vi "Ext.vi"(8 "error in (no error)":errorcluster, 9 "Val":variant, 10 "Tag":u16, 11 "Square in":refnum<class "Rigol DG822 Square.lvclass">) -> (0 "error out":errorcluster, 1 "Parsed":variant, 3 "Square out":refnum<class "Rigol DG822 Square.lvclass">)   [LabVIEW 2021, in "Rigol DG822 UI.lvlib" / "Rigol DG822 Square.lvlib" / "Rigol DG822 Square.lvclass"]
uses:
  Rigol DG822 Square.lvclass
  Rigol DG822 UI/lib/controls.llb/WaveformExtCall.ctl
  Rigol DG822 UI/lib/controls.llb/WaveformParamTags.ctl
  Rigol DG822 Square.lvclass/Rigol DG822 Square.ctl
  Rigol DG822 UI/lib/controls.llb/AllWaveformDataCluster.ctl
  Rigol DG822 UI/lib/controls.llb/DataCluster.ctl
  Rigol DG822 UI/lib/controls.llb/FT Controls Cluster.ctl
  Rigol DG822 UI/lib/controls.llb/String Indicators Cluster.ctl
  General/Files/lvlibp/Actors.lvlibp/Actors/Actors/Actors.lvclass
  D:/LabVIEW/General/Files/lvlibp/Actors.lvlibp/Actors/Actors/Actors.lvclass
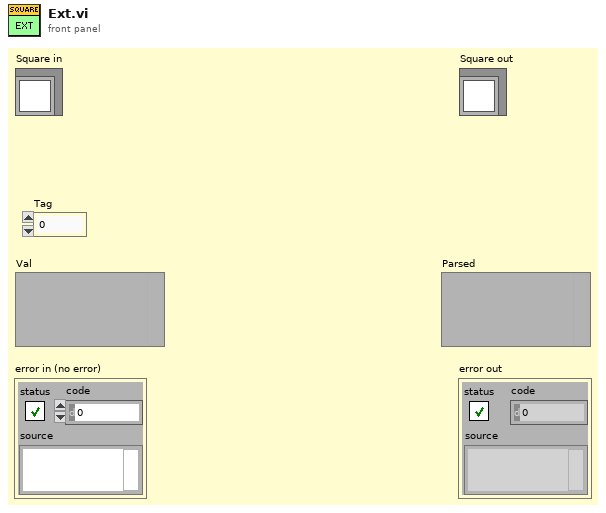
[diagram p1: front panel]
types:
  T1 = typedef "WaveformExtCall.ctl" = enum16{"Freq", "Period", "Ampl", "HighL", "Offset", "LowL", "Phase", "Duty", "Width", "RisEdge", "FallEdge", "Home", "InitData"}
  T2 = typedef "AllWaveformDataCluster.ctl" = cluster{"Data":T3, "F/T Ctrls":T4, "String Indcs":T5}
  T3 = typedef "DataCluster.ctl" = cluster{"Freq":cluster{"Freq":dbl, "FreqUnit":enum32{"No Selection", "MHz", "kHz", "Hz", "mHz", "uHz"}, "FreqUnitPrcs":dbl}, "Period":cluster{"Period":dbl, "PeriodUnit":enum32{"No Selection", "s", "ms", "us", "ns"}, "PeriodUnitPrcs":dbl}, "Ampl":cluster{"Ampl":dbl, "AmplUnit":enum32{"No Selection", "Vpp", "mVpp"}, "AmplUnitPrcs":dbl}, "HighL":cluster{"HighL":dbl, "HighLUnit":enum32{"No Selection", "V", "mV"}, "HighLUnitPrcs":dbl}, "Offset":cluster{"Offset":dbl, "OffsetUnit":enum32{"No Selection", "Vdc", "mVdc"}, "OffsetUnitPrcs":dbl}, "LowL":cluster{"LowL":dbl, "LowLUnit":enum32{"No Selection", "V", "mV"}, "LowLUnitPrcs":dbl}, "Phase":cluster{"Phase":dbl, "PhaseUnit":enum32{"°"}, "PhaseUnitPrcs":dbl}, "Duty":cluster{"Duty":dbl, "DutyUnit":enum32{"%"}, "DutyUnitPrcs":dbl}, "Width":cluster{"Width":dbl, "WidthUnit":enum32{"No Selection", "s", "ms", "us", "ns"}, "WidthUnitPrcs":dbl}, "RisEdge":cluster{"RisEdge":dbl, "RisEdgeUnit":enum32{"No Selection", "s", "ms", "us", "ns"}, "RisEdgeUnitPrcs":dbl}, "FallEdge":cluster{"FallEdge":dbl, "FallEdgeUnit":enum32{"No Selection", "s", "ms", "us", "ns"}, "FallEdgeUnitPrcs":dbl}}
  T4 = typedef "FT Controls Cluster.ctl" = cluster{"Freq/Period":bool, "Ampl/HighL":bool, "Offset/LowL":bool, "Duty/Width":bool}
  T5 = typedef "String Indicators Cluster.ctl" = cluster{"Freq-Period":string, "Ampl-HighL":string, "Offset-LowL":string, "Phase":string, "Duty-Width":string, "RisEdge":string, "FallEdge":string}
  T6 = typedef "WaveformParamTags.ctl" = enum16{"Freq", "Period", "Ampl", "HighL", "Offset", "LowL", "Phase", "Duty", "Width", "RisEdge", "FallEdge"}
  T7 = cluster{"Duty":dbl, "DutyUnit":enum32{"%"}, "DutyUnitPrcs":dbl}
  T8 = cluster{"Freq":dbl, "FreqUnit":enum32{"No Selection", "MHz", "kHz", "Hz", "mHz", "uHz"}, "FreqUnitPrcs":dbl}
  T9 = cluster{"Period":dbl, "PeriodUnit":enum32{"No Selection", "s", "ms", "us", "ns"}, "PeriodUnitPrcs":dbl}
  T10 = cluster{"Freq":cluster{"Freq":dbl, "FreqUnit":enum32{"No Selection", "MHz", "kHz", "Hz", "mHz", "uHz"}, "FreqUnitPrcs":dbl}, "Period":cluster{"Period":dbl, "PeriodUnit":enum32{"No Selection", "s", "ms", "us", "ns"}, "PeriodUnitPrcs":dbl}, "Duty":cluster{"Duty":dbl, "DutyUnit":enum32{"%"}, "DutyUnitPrcs":dbl}}
  T11 = cluster{"Ampl":dbl, "AmplUnit":enum32{"No Selection", "Vpp", "mVpp"}, "AmplUnitPrcs":dbl}
  T12 = cluster{"HighL":dbl, "HighLUnit":enum32{"No Selection", "V", "mV"}, "HighLUnitPrcs":dbl}
  T13 = cluster{"Offset":dbl, "OffsetUnit":enum32{"No Selection", "Vdc", "mVdc"}, "OffsetUnitPrcs":dbl}
  T14 = cluster{"LowL":dbl, "LowLUnit":enum32{"No Selection", "V", "mV"}, "LowLUnitPrcs":dbl}
  T15 = cluster{"Ampl":cluster{"Ampl":dbl, "AmplUnit":enum32{"No Selection", "Vpp", "mVpp"}, "AmplUnitPrcs":dbl}, "HighL":cluster{"HighL":dbl, "HighLUnit":enum32{"No Selection", "V", "mV"}, "HighLUnitPrcs":dbl}, "Offset":cluster{"Offset":dbl, "OffsetUnit":enum32{"No Selection", "Vdc", "mVdc"}, "OffsetUnitPrcs":dbl}, "LowL":cluster{"LowL":dbl, "LowLUnit":enum32{"No Selection", "V", "mV"}, "LowLUnitPrcs":dbl}}
  T16 = cluster{"Phase":dbl, "PhaseUnit":enum32{"°"}, "PhaseUnitPrcs":dbl}
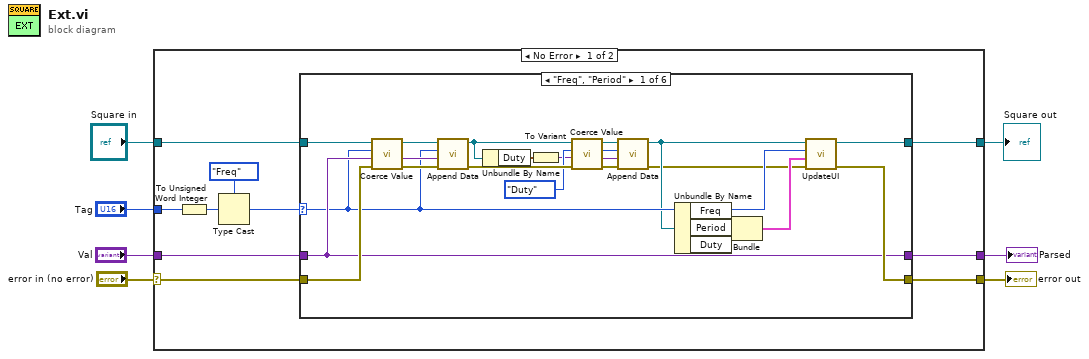
[diagram p0: block diagram]
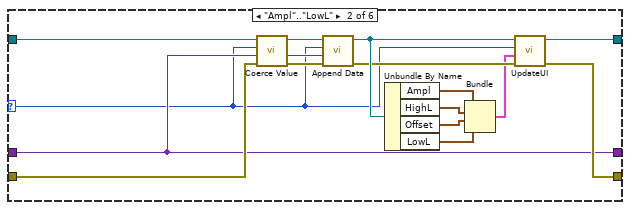
[diagram p2: hidden frame]
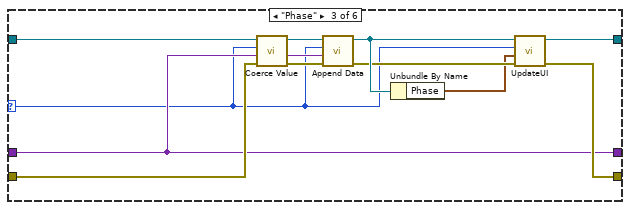
[diagram p3: hidden frame]
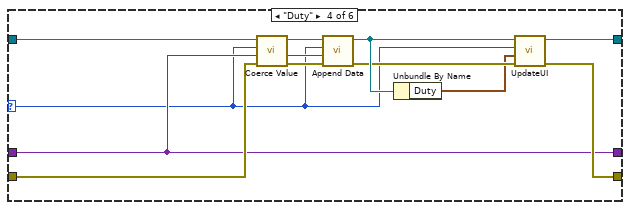
[diagram p4: hidden frame]
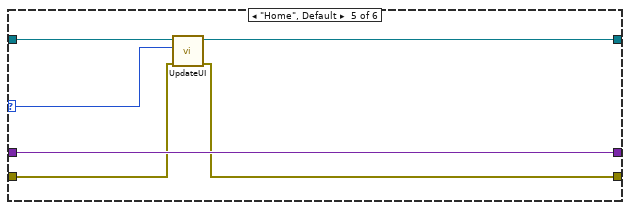
[diagram p5: hidden frame]
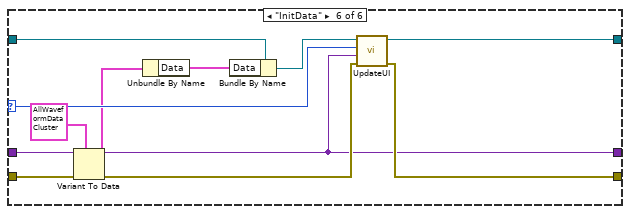
[diagram p6: hidden frame]
diagram:
  n1 = case shown="No Error" "error in (no error)" {
    selector: "error in (no error)" -> [w10 w99]
    tunnel: [w12 w98] -> w3
    tunnel: "Square in" -> [w13 w98]
    tunnel: "Tag" -> [w16 _]
    tunnel: "Val" -> [w15 _]
    tunnel: [w11 _] -> w2
    tunnel: [w9 w99] -> w1
    frame No Error {
      n2 = To Unsigned Word Integer(number=w16) -> (unsigned 16bit integer=w17:u16)
      n3 = Type Cast(type=WaveformExtCall."Freq" ("Enum"), x=w17) -> (*(type *) &x=w14:T1)
      n4 = case shown="\"Freq\", \"Period\"" w14 {
        selector: w14 -> [w32 w46 w58 w70 w84 w96]
        tunnel: w15 -> [w35 w50 w62 w74 w83 w90]
        tunnel: w13 -> [w37 w52 w64 w76 w86 w94]
        tunnel: [w40 w56 w68 w80 w85 w97] -> w12
        tunnel: [w35 w50 w62 w74 w83 w90] -> w11
        tunnel: w10 -> [w36 w51 w63 w75 w82 w92]
        tunnel: [w39 w55 w67 w79 w81 w95] -> w9
        frame "Freq", "Period" {
          w24 = WaveformParamTags."Duty" ("ParamTags")
          n5 = call-dynamic "Coerce Value.vi"("error in (no error)"=w36, "Value"=w35, "ParamTags"=w32, "Rigol DG822 Square in"=w37) -> ("error out"=w33:errorcluster, "Coerced Value"=w34:variant, "Rigol DG822 Square out"=w38:refnum<class "Rigol DG822 Square.lvclass">)  [unwired: 5 in]
          n6 = call-dynamic "Append Data.vi"("error in (no error)"=w33, "Data"=w34, "ParamTags"=w32, "Rigol DG822 Square in"=w38) -> ("error out"=w25:errorcluster, "Rigol DG822 Square out"=w21:refnum<class "Rigol DG822 Square.lvclass">)  [unwired: 6 in]
          n7 = Unbundle By Name(w21) -> ("Duty"=w20:T7)
          n8 = To Variant(anything=w20) -> (Variant=w19:variant)
          n9 = call-dynamic "Coerce Value.vi"("error in (no error)"=w25, "Value"=w19, "ParamTags"=w24, "Rigol DG822 Square in"=w21) -> ("error out"=w18:errorcluster, "Coerced Value"=w27:variant, "Rigol DG822 Square out"=w26:refnum<class "Rigol DG822 Square.lvclass">)  [unwired: 5 in]
          n10 = call-dynamic "Append Data.vi"("error in (no error)"=w18, "Data"=w27, "ParamTags"=w24, "Rigol DG822 Square in"=w26) -> ("error out"=w22:errorcluster, "Rigol DG822 Square out"=w23:refnum<class "Rigol DG822 Square.lvclass">)  [unwired: 6 in]
          n11 = Unbundle By Name(w23) -> ("Freq"=w30:T8, "Period"=w29:T9, "Duty"=w28:T7)
          n12 = Bundle("Freq"=w30, "Period"=w29, "Duty"=w28) -> (w31:T10)  [unwired: 1 in]
          n13 = call "UpdateUI.vi"("error in (no error)"=w22, "Data"=w31, "Type"=w32, "Recursive in"=w23) -> ("error out"=w39:errorcluster, "Recursive out"=w40:refnum<class "Rigol DG822 Square.lvclass">)  [unwired: 6 in]
        }
        frame "Ampl".."LowL" {
          n14 = call-dynamic "Coerce Value.vi"("error in (no error)"=w51, "Value"=w50, "ParamTags"=w46, "Rigol DG822 Square in"=w52) -> ("error out"=w48:errorcluster, "Coerced Value"=w49:variant, "Rigol DG822 Square out"=w53:refnum<class "Rigol DG822 Square.lvclass">)  [unwired: 5 in]
          n15 = call-dynamic "Append Data.vi"("error in (no error)"=w48, "Data"=w49, "ParamTags"=w46, "Rigol DG822 Square in"=w53) -> ("error out"=w47:errorcluster, "Rigol DG822 Square out"=w54:refnum<class "Rigol DG822 Square.lvclass">)  [unwired: 6 in]
          n16 = Unbundle By Name(w54) -> ("Ampl"=w45:T11, "HighL"=w42:T12, "Offset"=w41:T13, "LowL"=w43:T14)
          n17 = Bundle("Ampl"=w45, "HighL"=w42, "Offset"=w41, "LowL"=w43) -> (w44:T15)  [unwired: 1 in]
          n18 = call "UpdateUI.vi"("error in (no error)"=w47, "Data"=w44, "Type"=w46, "Recursive in"=w54) -> ("error out"=w55:errorcluster, "Recursive out"=w56:refnum<class "Rigol DG822 Square.lvclass">)  [unwired: 6 in]
        }
        frame "Phase" {
          n19 = call-dynamic "Coerce Value.vi"("error in (no error)"=w63, "Value"=w62, "ParamTags"=w58, "Rigol DG822 Square in"=w64) -> ("error out"=w60:errorcluster, "Coerced Value"=w61:variant, "Rigol DG822 Square out"=w65:refnum<class "Rigol DG822 Square.lvclass">)  [unwired: 5 in]
          n20 = call-dynamic "Append Data.vi"("error in (no error)"=w60, "Data"=w61, "ParamTags"=w58, "Rigol DG822 Square in"=w65) -> ("error out"=w59:errorcluster, "Rigol DG822 Square out"=w66:refnum<class "Rigol DG822 Square.lvclass">)  [unwired: 6 in]
          n21 = Unbundle By Name(w66) -> ("Phase"=w57:T16)
          n22 = call "UpdateUI.vi"("error in (no error)"=w59, "Data"=w57, "Type"=w58, "Recursive in"=w66) -> ("error out"=w67:errorcluster, "Recursive out"=w68:refnum<class "Rigol DG822 Square.lvclass">)  [unwired: 6 in]
        }
        frame "Duty" {
          n23 = call-dynamic "Coerce Value.vi"("error in (no error)"=w75, "Value"=w74, "ParamTags"=w70, "Rigol DG822 Square in"=w76) -> ("error out"=w72:errorcluster, "Coerced Value"=w73:variant, "Rigol DG822 Square out"=w77:refnum<class "Rigol DG822 Square.lvclass">)  [unwired: 5 in]
          n24 = call-dynamic "Append Data.vi"("error in (no error)"=w72, "Data"=w73, "ParamTags"=w70, "Rigol DG822 Square in"=w77) -> ("error out"=w71:errorcluster, "Rigol DG822 Square out"=w78:refnum<class "Rigol DG822 Square.lvclass">)  [unwired: 6 in]
          n25 = Unbundle By Name(w78) -> ("Duty"=w69:T7)
          n26 = call "UpdateUI.vi"("error in (no error)"=w71, "Data"=w69, "Type"=w70, "Recursive in"=w78) -> ("error out"=w79:errorcluster, "Recursive out"=w80:refnum<class "Rigol DG822 Square.lvclass">)  [unwired: 6 in]
        }
        frame "Home", Default {
          n27 = call "UpdateUI.vi"("error in (no error)"=w82, "Type"=w84, "Recursive in"=w86) -> ("error out"=w81:errorcluster, "Recursive out"=w85:refnum<class "Rigol DG822 Square.lvclass">)  [unwired: 7 in]
        }
        frame "InitData" {
          n28 = Variant To Data(error in=w92, type=T2 {"Data"={"Freq"={"Freq"=1.0, "FreqUnit"=enum."kHz", "FreqUnitPrcs"=9.0}, "Period"={"Period"=1.0, "PeriodUnit"=enum."ms", "PeriodUnitPrcs"=7.0}, "Ampl"={"Ampl"=5.0, "AmplUnit"=enum."Vpp", "AmplUnitPrcs"=4.0}, "HighL"={"HighL"=2.5, "HighLUnit"=enum."V", "HighLUnitPrcs"=4.0}, "Offset"={"Offset"=0.0, "OffsetUnit"=enum."Vdc", "OffsetUnitPrcs"=4.0}, "LowL"={"LowL"=-2.5, "LowLUnit"=enum."V", "LowLUnitPrcs"=4.0}, "Phase"={"Phase"=0.0, "PhaseUnit"=enum."°", "PhaseUnitPrcs"=3.0}, "Duty"={"Duty"=50.0, "DutyUnit"=enum."%", "DutyUnitPrcs"=3.0}, "Width"={"Width"=500.0, "WidthUnit"=enum."us", "WidthUnitPrcs"=4.0}, "RisEdge"={"RisEdge"=10.0, "RisEdgeUnit"=enum."ns", "RisEdgeUnitPrcs"=1.0}, "FallEdge"={"FallEdge"=10.0, "FallEdgeUnit"=enum."ns", "FallEdgeUnitPrcs"=1.0}}, "F/T Ctrls"={"Freq/Period"=FALSE, "Ampl/HighL"=FALSE, "Offset/LowL"=FALSE, "Duty/Width"=FALSE}, "String Indcs"={"Freq-Period"="1.000,000,000 kHz", "Ampl-HighL"="5.000,0 Vpp", "Offset-LowL"="0.000,0 Vdc", "Phase"="0.000 °", "Duty-Width"="50.000 %", "RisEdge"="10.0 ns", "FallEdge"="10.0 ns"}} ("Params Data"), Variant=w90) -> (data=w88:T2, error out=w91:errorcluster)
          n29 = Unbundle By Name(w88) -> ("Data"=w89:T3)
          n30 = Bundle By Name(cluster=w94, "Data"=w89) -> (w93:refnum<class "Rigol DG822 Square.lvclass">)
          n31 = call "UpdateUI.vi"("error in (no error)"=w91, "Data"=w90, "Type"=w96, "Recursive in"=w93) -> ("error out"=w95:errorcluster, "Recursive out"=w97:refnum<class "Rigol DG822 Square.lvclass">)  [unwired: 6 in]
        }
      }
    }
    frame Error {
    }
  }
  "error out" <- w1
  "Square out" <- w3
  "Parsed" <- w2
